vi "cursor window logic.vi"(4 "h. offset":dbl, 6 "CursIdx":i32, 7 "cursor window action":T1=enum."check", 8 "window":dbl=nan, 9 "center":dbl=nan, 10 "cursor bracket in":refnum<vi>, 11 "cursor bracket in":T2={"left"=2044.0881763527054, "right "=2126.7657992565055, "center"=2085.4269878046052, "window"=82.67762290380006, "cursors"=[], "relative"=0, "absolute"=0, "fixed vertical offset"=2421.6740576496672, "vertical offset"=2421.6740576496672, "skew"=2421.6740576496672, "default window frac"=2421.6740576496672, "kind"=enum."fancy", "skew.left"=2.0, "skew.right"=0.0, "Plot ref"=refnum, "wing order"=enum."back"}) -> (2 "reference out":refnum<vi>, 3 "cursor window out":T2={"left"=2044.0881763527054, "right "=2126.7657992565055, "center"=2085.4269878046052, "window"=82.67762290380006, "cursors"=[], "relative"=0, "absolute"=0, "fixed vertical offset"=2421.6740576496672, "vertical offset"=2421.6740576496672, "skew"=2421.6740576496672, "default window frac"=2421.6740576496672, "kind"=enum."fancy", "skew.left"=2.0, "skew.right"=0.0, "Plot ref"=refnum, "wing order"=enum."back"})   [LabVIEW 2014]
uses:
  cursor winow.ctl
  cursor window action.ctl
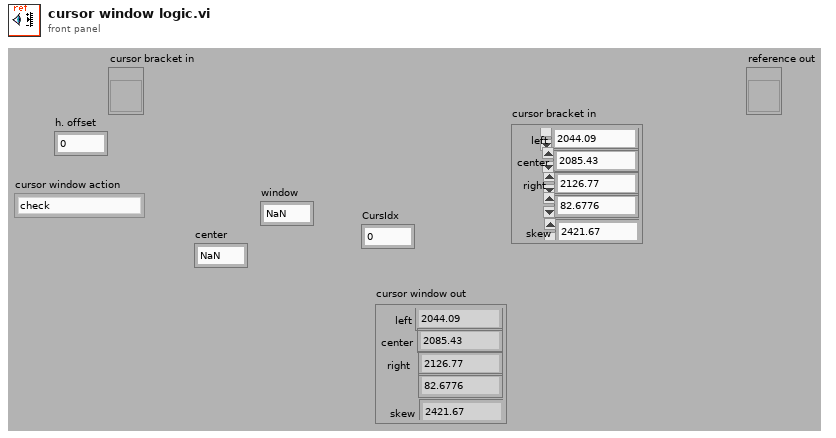
[diagram p1: front panel]
types:
  T1 = typedef "cursor window action.ctl" = enum16{"balance", "h. offset change", "cursor moves", "change center", "change window", "init", "check", "reset", "set y to middle", "idle", "-write all Y", "-write left.X", "-write center.X", "-write right.X", "-write all X", "-change center", "-change window", "-change skew", "-read cursor 2", "-read cursor 1", "-read cursor 0", "-read all cursors", "-reset", "-read plot scale", "-set y to middle", "-Q: center.Y is visible", "-Q: window is visible", "-parse center.Y", "-right left from center", "-left move", "-right move", "-set center.Y", "-empty", "-set cursors to default", "-check", "-write center.Y", "-copy cursor 1", "-copy cursor 0", "-copy cursor 2", "move right", "move left", "shrink", "broaden", "skew up", "skew down", "-write plot scale", "zoom X", "change cen&win", "zoom to all data"}
  T2 = typedef "cursor winow.ctl" = cluster{"left":dbl, "right ":dbl, "center":dbl, "window":dbl, "cursors":i32[], "relative":i32, "absolute":i32, "fixed vertical offset":dbl, "vertical offset":dbl, "skew":dbl, "default window frac":dbl, "kind":enum16{"symmetric", "skewed", "fancy"}, "skew.left":dbl, "skew.right":dbl, "Plot ref":refnum<vi>, "wing order":enum16{"forw", "back"}}
  T3 = cluster{"left":dbl, "right ":dbl, "center":dbl, "window":dbl, "cursors":i32[], "relative":i32, "absolute":i32, "fixed vertical offset":dbl, "vertical offset":dbl, "skew":dbl, "default window frac":dbl, "kind":enum16{"symmetric", "skewed", "fancy"}, "skew.left":dbl, "skew.right":dbl, "Plot ref":refnum<vi>, "wing order":enum16{"forw", "back"}}
  T4 = typedef "LVCursorListTypeDef.ctl" = cluster{"Name":string, "Color":u32, "Style":u8, "Point Style":u8, "Name Visible":bool, "Allow Drag":bool, "Cursor Mode":u32, "Plot":i32, "Index":i32, "Position":cluster{"X":dbl, "Y":dbl}, "X Scale":u32, "Y Scale":u32, "Watch Plots":i32[], "Watch All Plots":bool, "Plot Area":i32, "Label Offset":cluster{"X":dbl, "Y":dbl}}[]
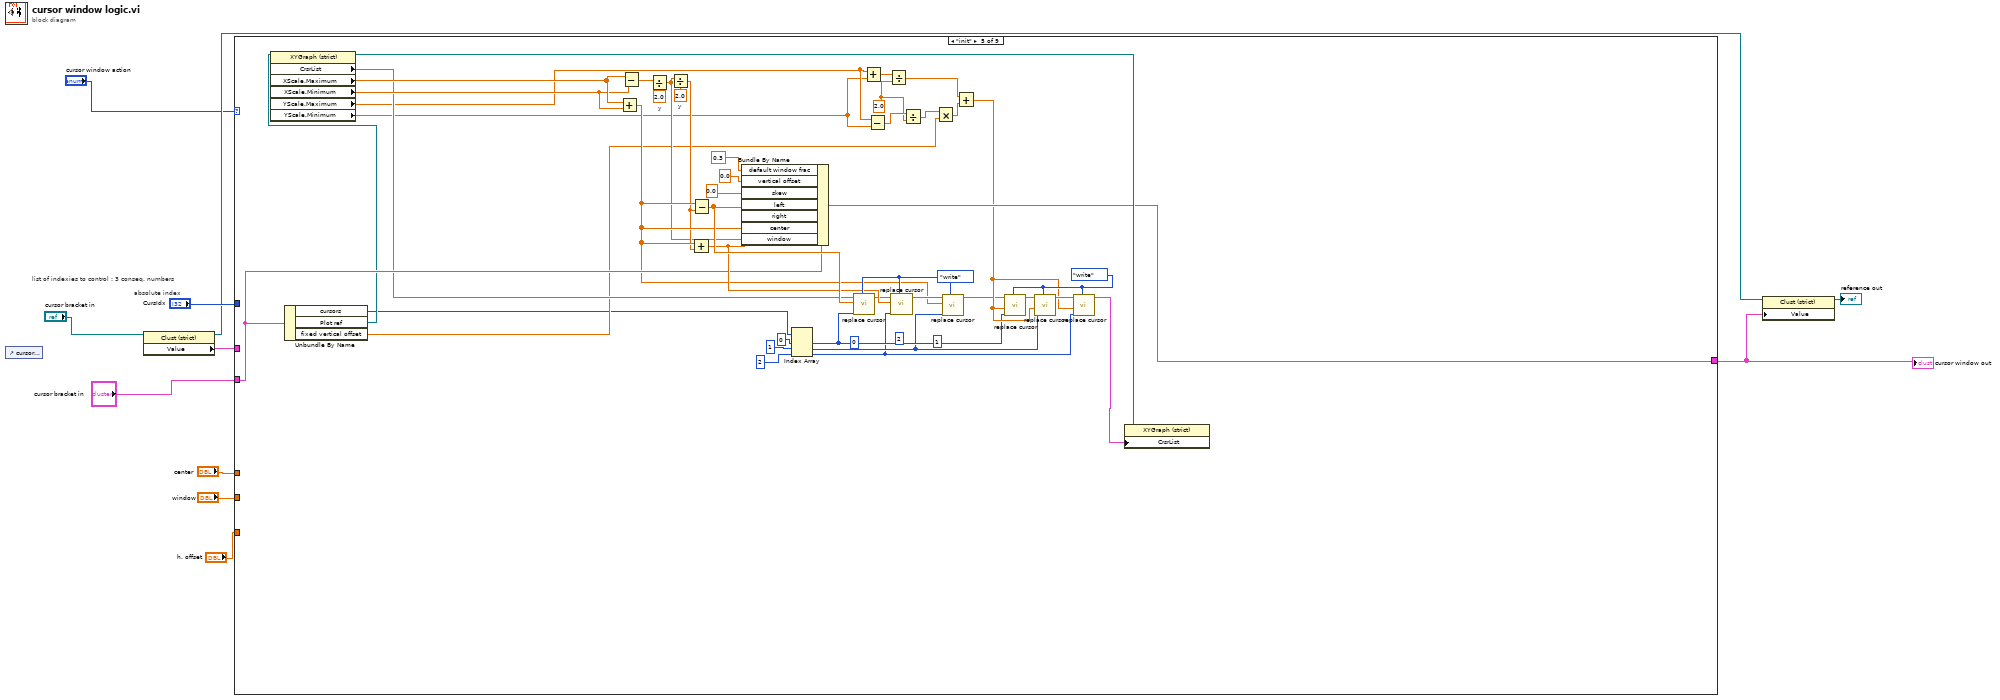
[diagram p0: block diagram]
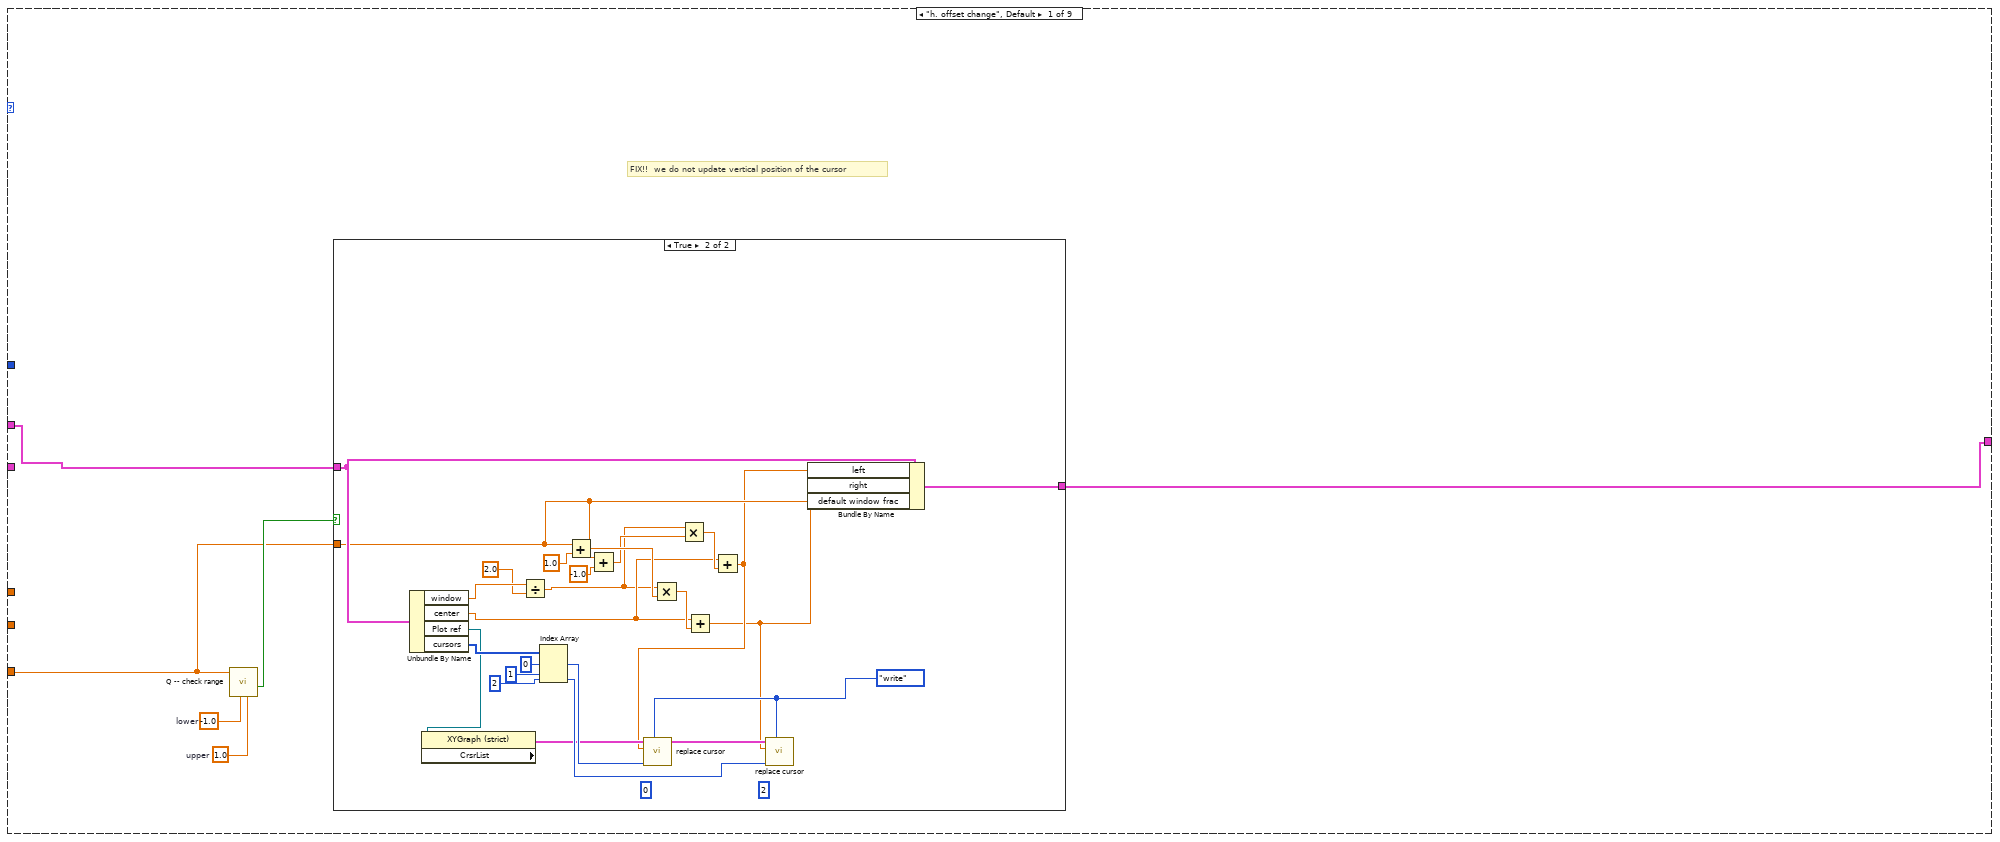
[diagram p2: hidden frame]
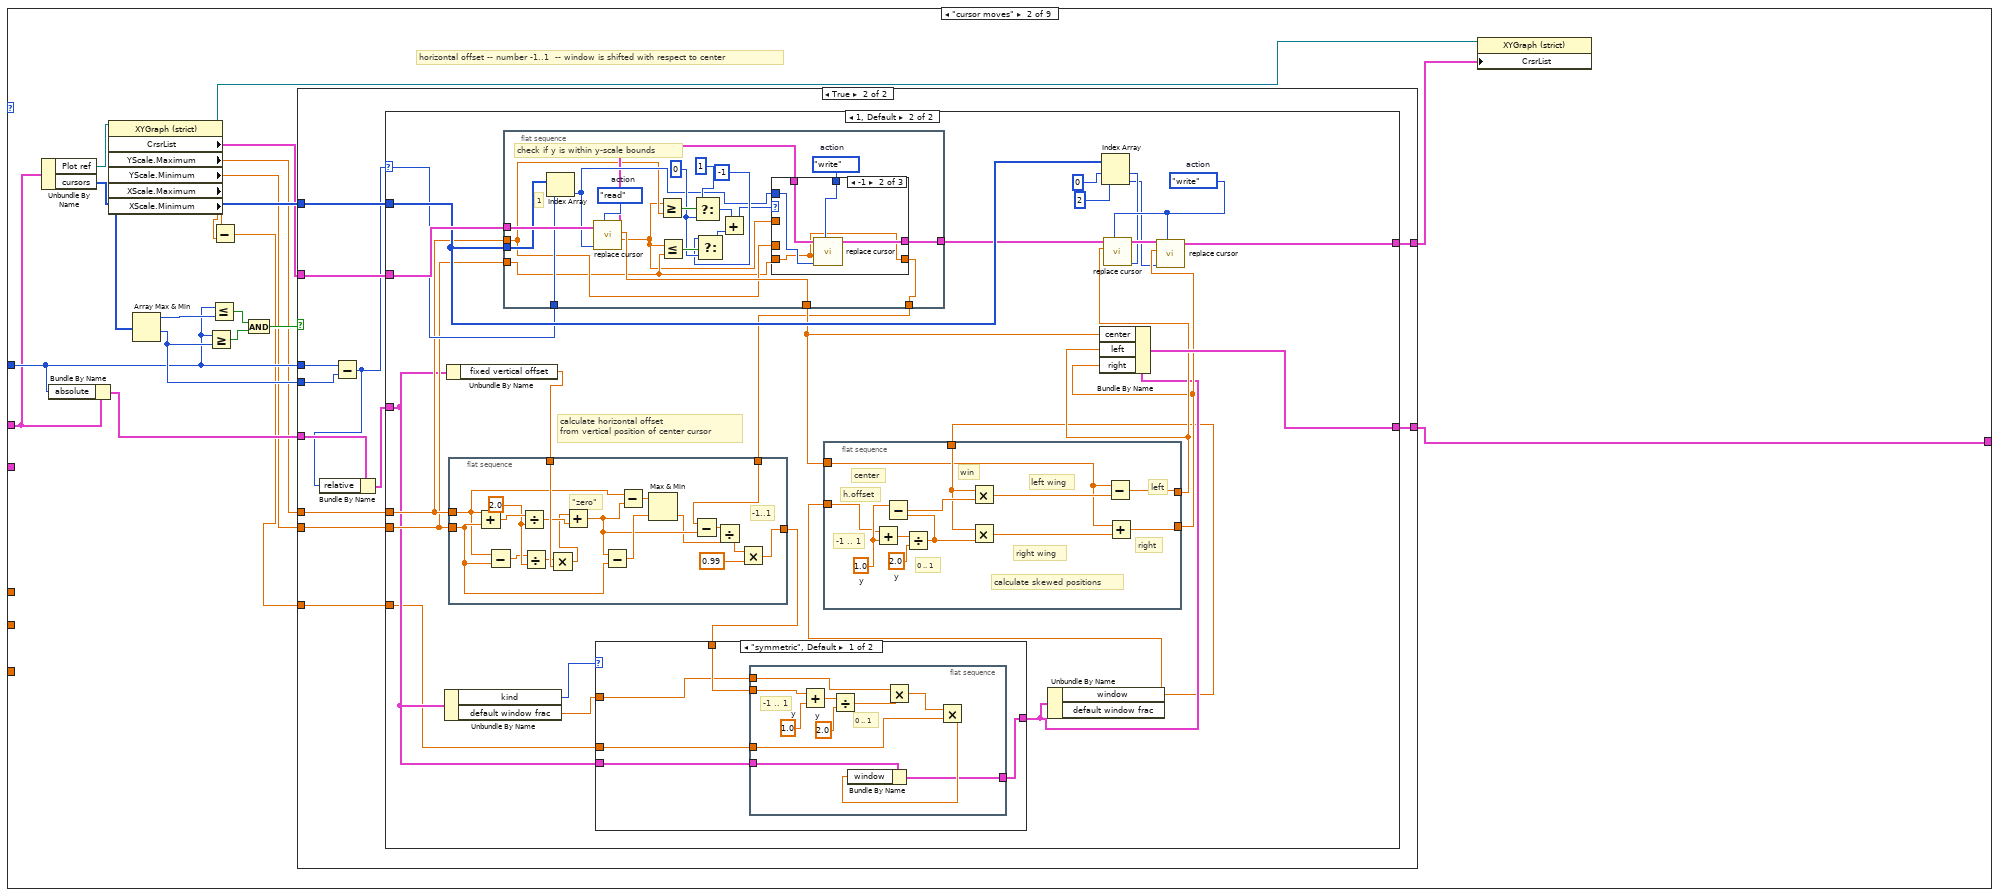
[diagram p4: hidden frame]
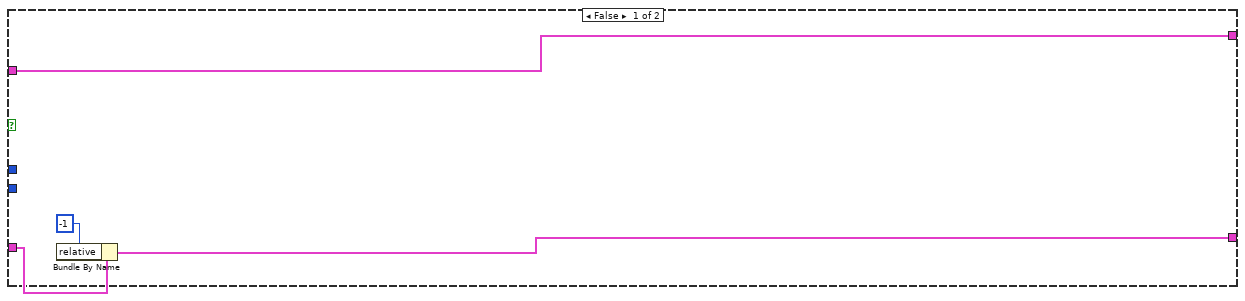
[diagram p5: hidden frame]
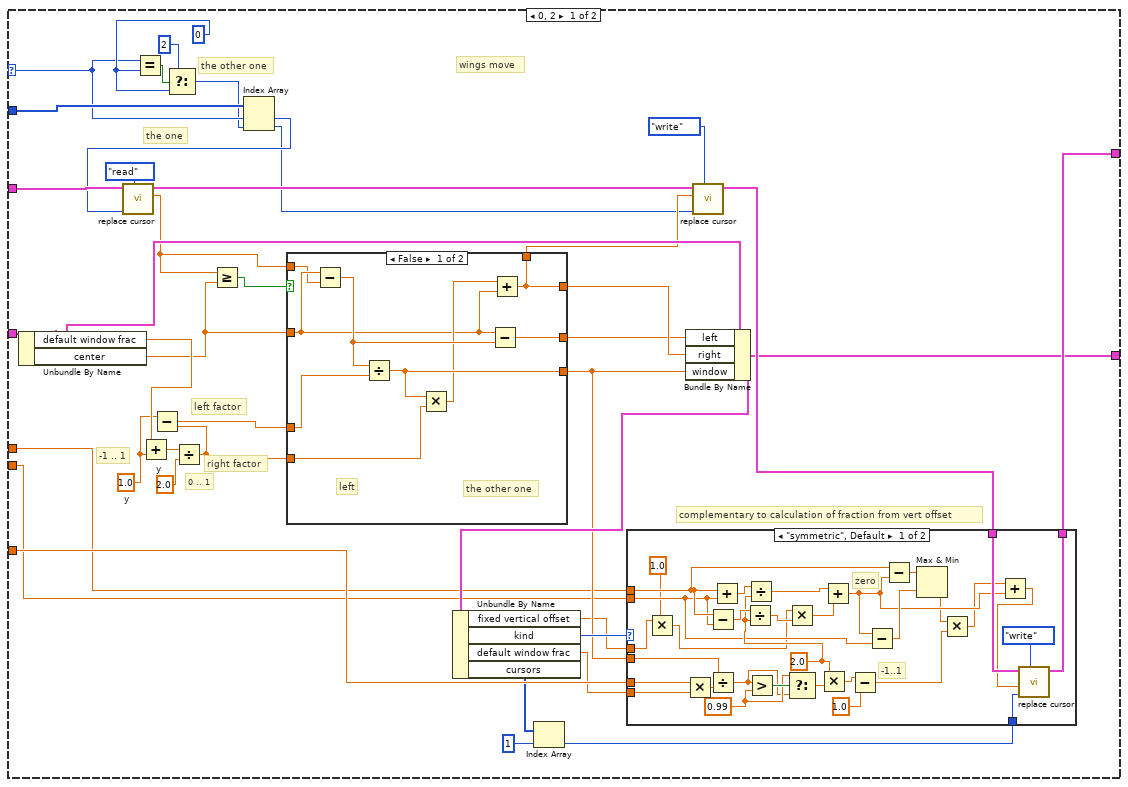
[diagram p6: hidden frame]
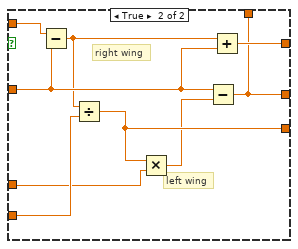
[diagram p8: hidden frame]
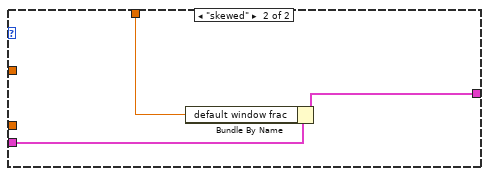
[diagram p9: hidden frame]
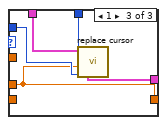
[diagram p11: hidden frame]
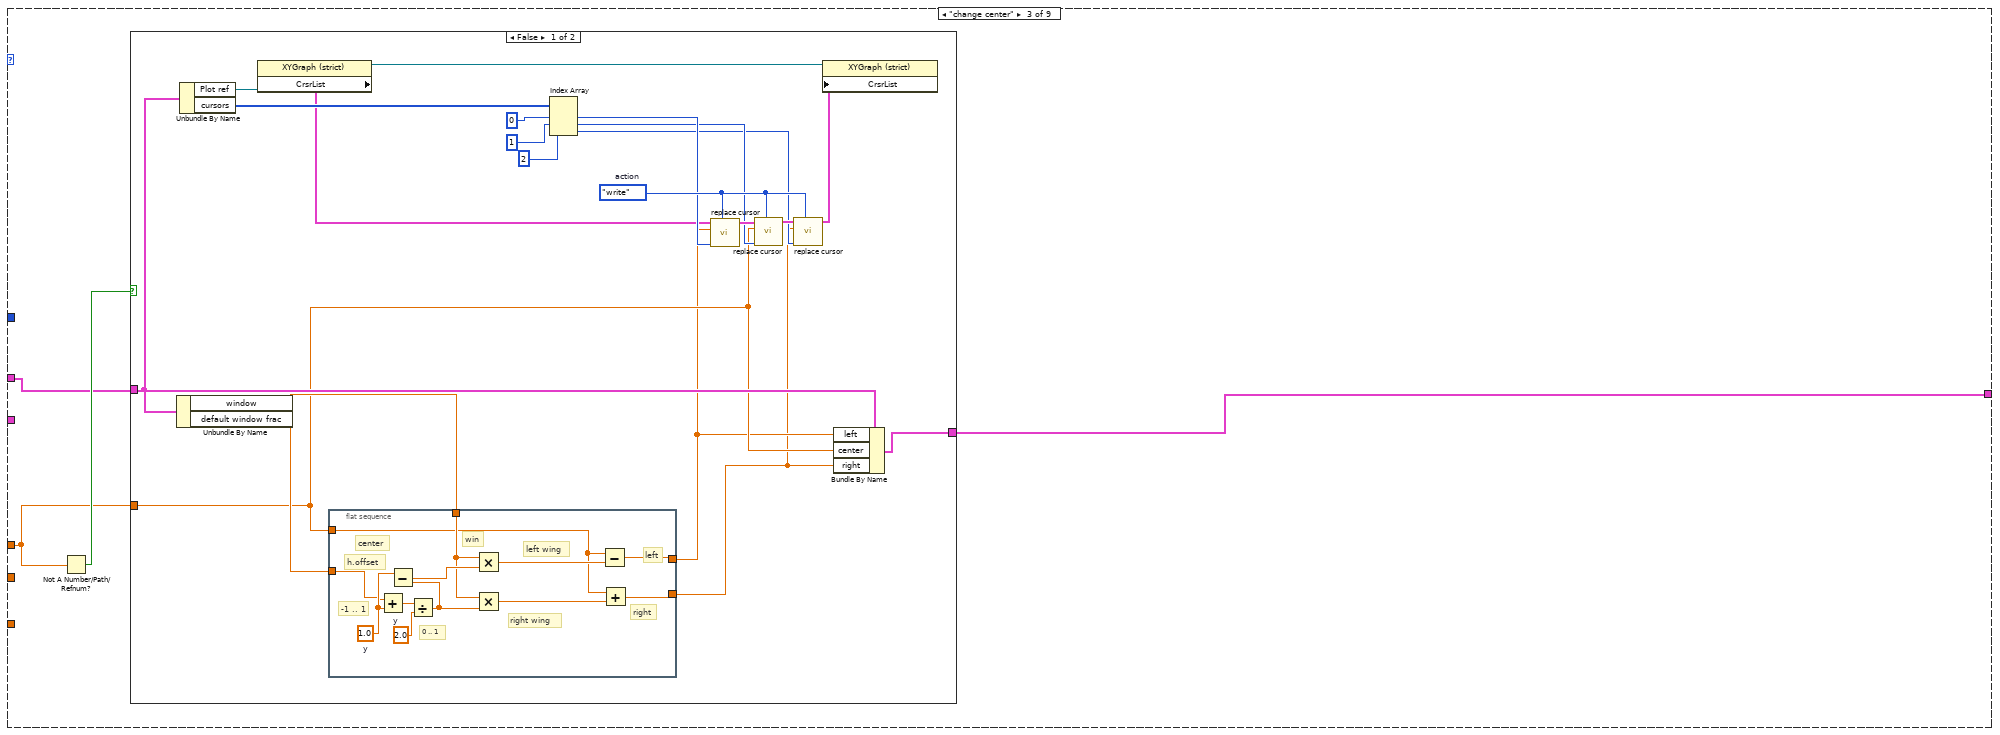
[diagram p12: hidden frame]
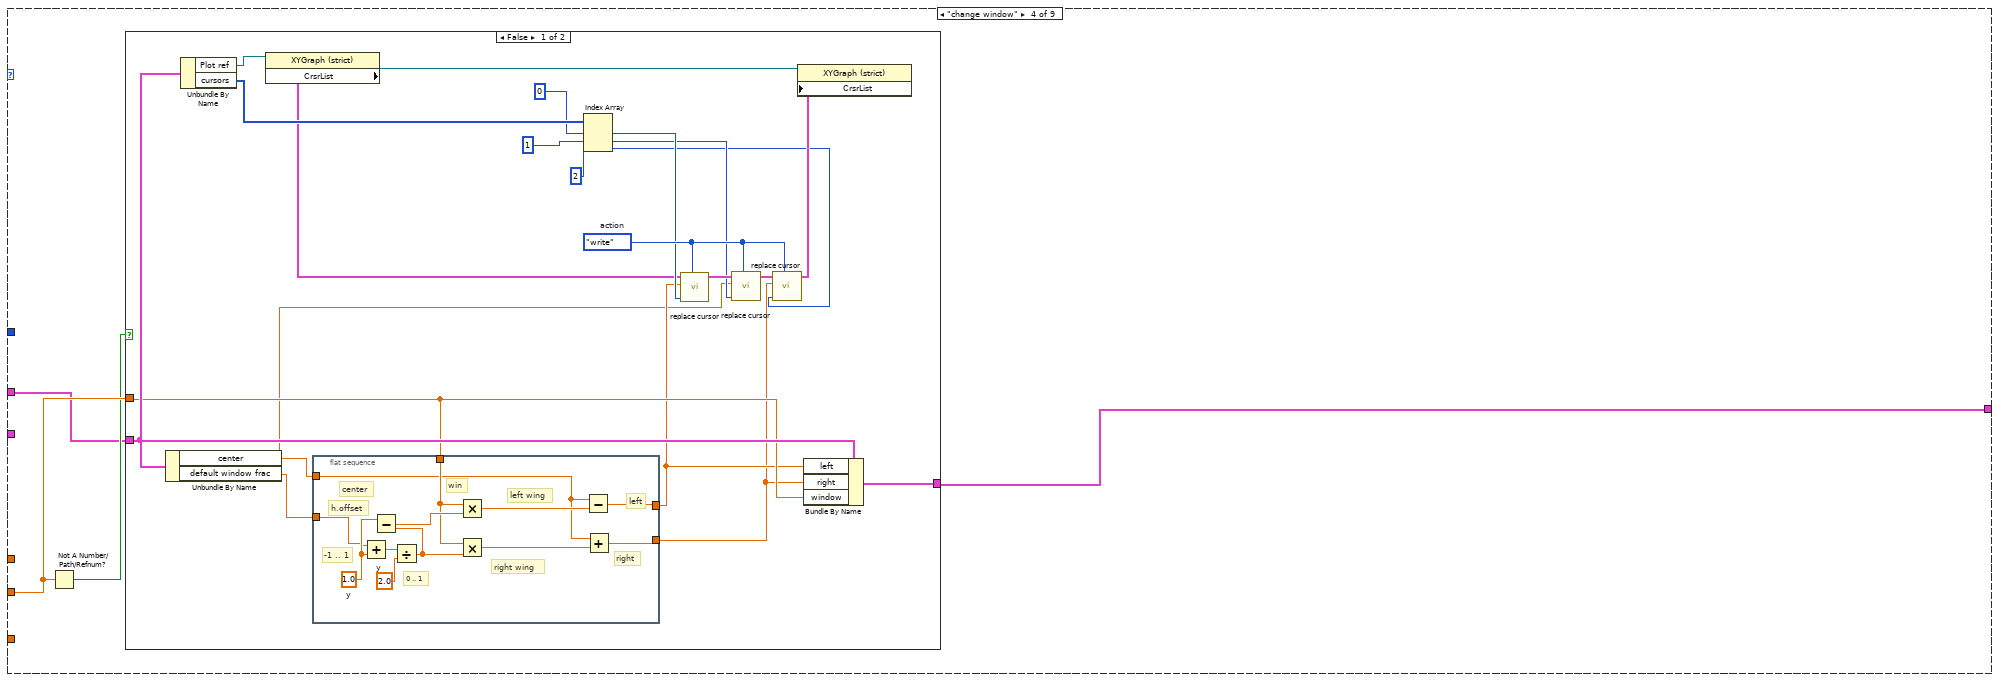
[diagram p14: hidden frame]
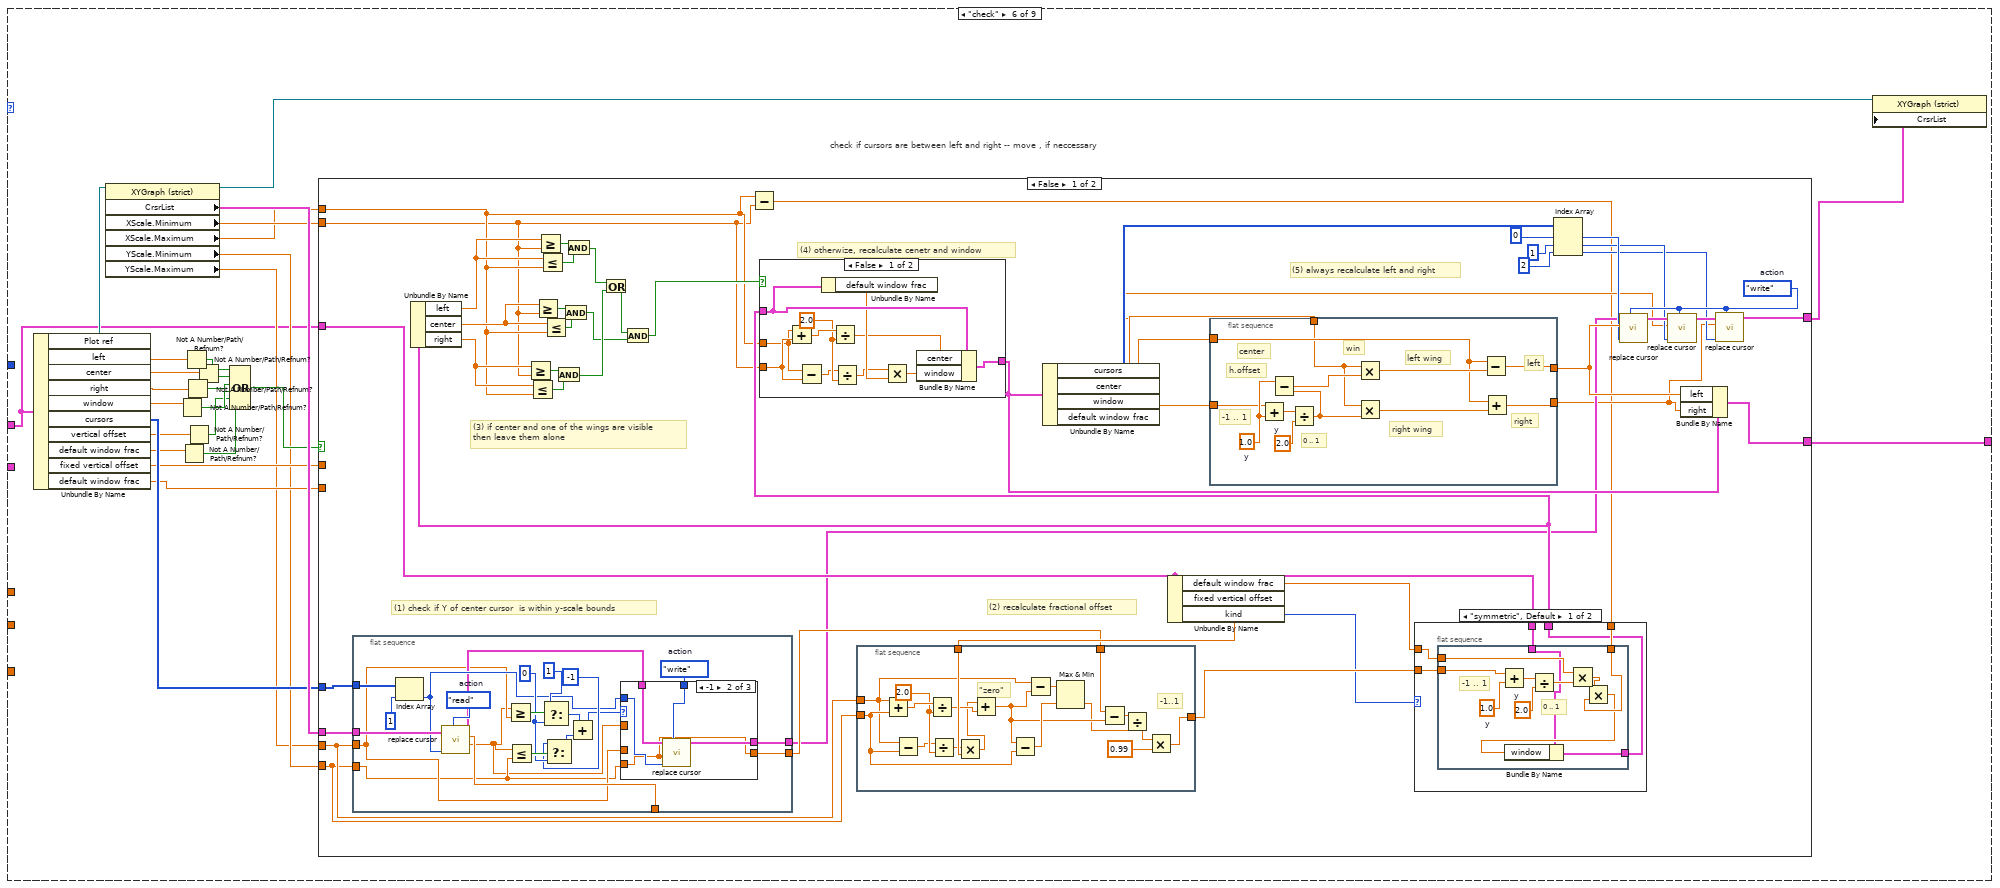
[diagram p16: hidden frame]
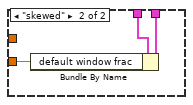
[diagram p17: hidden frame]
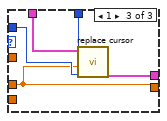
[diagram p19: hidden frame]
diagram:
  # "list of indexies to control : 3 conseq. numbers"
  # "absolute index"
  n1 = control-ref of="cursor bracket in"() -> ()  [unwired: 1 out]
  n2 = property class="Clust (strict)"(reference="cursor bracket in") -> (reference out=w6:refnum<vi>, "Value"=w7:T3)  [unwired: 1 in, 1 out]
  n3 = case shown="\"init\"" "cursor window action" {
    tunnel: "cursor bracket in" -> [_ _ _ _ w385 _ _ _ _]
    tunnel: [w12 w50 w280 w318 w386 w419 w605 w636 w661] -> w5
    tunnel: "CursIdx" -> [_ w56 _ _ _ _ _ _ _]
    tunnel: "center" -> [_ _ w278 _ _ _ _ _ _]
    tunnel: "window" -> [_ _ _ w317 _ _ _ _ _]
    tunnel: w7 -> [w17 w44 w277 w315 _ w396 w603 w636 w661]
    tunnel: "h. offset" -> [w13 _ _ _ _ _ _ _ _]
    frame "h. offset change", Default {
      w15 = 1.0  # upper
      w16 = -1.0  # lower
      # "FIX!!  we do not update vertical position of the cursor"
      n4 = call "Q -- check range.vi"("upper"=w15, "lower"=w16, "number"=w13) -> ("in range?"=w14:bool)  [unwired: 4 in, 4 out]
      n5 = case shown="True" w14 {
        tunnel: w17 -> [w18 w43]
        tunnel: w13 -> [_ w37]
        tunnel: [w18 w19] -> w12
        frame False {
        }
        frame True {
          w25 = enum16{"", "read", "write"}."write" ("Enum")
          (unwired) 2 ("cursor index")
          (unwired) 0 ("cursor index")
          n6 = Unbundle By Name(w43) -> ("window"=w42:dbl, "center"=w34:dbl, "Plot ref"=w23:refnum<vi>, "cursors"=w24:i32[])
          n7 = property class="XYGraph (strict)"(reference=w23) -> ("CrsrList"=w22:T4)  [unwired: 1 in, 2 out]
          n8 = Divide(x=w42, y=2.0) -> (x/y=w32:dbl)
          n9 = Index Array(array=w24, index #1=0 ("index"), index #2=1 ("index"), index #3=2 ("index")) -> (element #1=w28:i32, element #3=w27:i32)  [unwired: 1 out]
          n10 = Add(x=w37, y=1.0) -> (x+y=w36:dbl)
          n11 = Add(x=w37, y=-1.0) -> (x+y=w33:dbl)
          n12 = Multiply(x=w32, y=w36) -> (x*y=w40:dbl)
          n13 = Multiply(x=w32, y=w33) -> (x*y=w35:dbl)
          n14 = Add(x=w34, y=w40) -> (x+y=w20:dbl)
          n15 = Add(x=w34, y=w35) -> (x+y=w21:dbl)
          n16 = call "replace cursor.vi"("action"=w25, "cursor index"=w28, "new X"=w21, "Cursor List in"=w22) -> ("Cursor List Out"=w26:T4)  [unwired: 5 in, 2 out]
          n17 = call "replace cursor.vi"("action"=w25, "cursor index"=w27, "new X"=w20, "Cursor List in"=w26) -> ()  [unwired: 5 in, 3 out]
          n18 = Bundle By Name(cluster=w43, "left"=w21, "right"=w20, "default window frac"=w37) -> (w19:T3)
        }
      }
    }
    frame "cursor moves" {
      # "horizontal offset -- number -1..1  -- window is shifted with respect to center"
      n19 = Unbundle By Name(w44) -> ("Plot ref"=w54:refnum<vi>, "cursors"=w55:i32[])
      n20 = Bundle By Name(cluster=w44, "absolute"=w56) -> (w57:T3)
      n21 = property on="Property Node" class="XYGraph (strict)"(reference=w54) -> (reference out=w51:refnum<vi>, "CrsrList"=w53:T4, "YScale.Maximum"=w49:dbl, "YScale.Minimum"=w48:dbl, "XScale.Maximum"=w47:dbl, "XScale.Minimum"=w46:dbl)  [unwired: 1 in, 1 out]
      n22 = Array Max & Min(array=w55) -> (max value=w62:i32, min value=w58:i32)  [unwired: 2 out]
      n23 = Greater Or Equal?(x=w56, y=w58) -> (x >= y?=w61:bool)
      n24 = Less Or Equal?(x=w56, y=w62) -> (x <= y?=w60:bool)
      n25 = Subtract(x=w47, y=w46) -> (x-y=w45:dbl)
      n26 = And(x=w60, y=w61) -> (x .and. y?=w59:bool)
      n27 = case shown="True" w59 {
        tunnel: w57 -> [w65 w72]
        tunnel: [w63 w78] -> w50
        tunnel: w53 -> [w66 w77]
        tunnel: [w66 w76] -> w52
        tunnel: w55 -> [_ w75]
        tunnel: w56 -> [_ w74]
        tunnel: w58 -> [_ w73]
        tunnel: w49 -> [_ w69]
        tunnel: w48 -> [_ w68]
        tunnel: w45 -> [_ w67]
        frame False {
          n28 = Bundle By Name(cluster=w65, "relative"=-1) -> (w63:T3)
        }
        frame True {
          n29 = Subtract(x=w74, y=w73) -> (x-y=w70:i32)
          n30 = Bundle By Name(cluster=w72, "relative"=w70) -> (w71:T3)
          n31 = case shown="1, Default" w70 {
            selector: w70 -> [w97 w186]
            tunnel: w77 -> [w116 w194]
            tunnel: w71 -> [w114 w174]
            tunnel: [w88 w193] -> w78
            tunnel: [w91 w190] -> w76
            tunnel: w75 -> [w110 w187]
            tunnel: w69 -> [w84 w179]
            tunnel: w68 -> [w83 w177]
            tunnel: w67 -> [w89 w168]
            frame 0, 2 {
              w99 = 0 ("y")
              w106 = 1.0  # y
              w109 = 2.0  # y
              # "complementary to calculation of fraction from vert offset"
              # "wings move"
              # "the one"
              # "the other one"
              # "left factor"
              # "right factor"
              # "0 .. 1"
              # "-1 .. 1"
              n32 = Unbundle By Name(w114) -> ("default window frac"=w107:dbl, "center"=w95:dbl)
              n33 = Equal?(x=w97, y=w99) -> (x = y?=w98:bool)
              n34 = Add(x=w107, y=w106) -> (x+y=w108:dbl)
              n35 = Select(t=2, s=w98, f=w99) -> (s? t:f=w94:i32)
              n36 = Divide(x=w108, y=w109) -> (x/y=w104:dbl)
              n37 = Subtract(x=w106, y=w104) -> (x-y=w102:dbl)
              n38 = Index Array(array=w110, index #1=w97, index #2=w94) -> (element #1=w111:i32, element #2=w93:i32)
              n39 = call "replace cursor.vi"("action"=enum16{"", "read", "write"}."read", "cursor index"=w111, "Cursor List in"=w116) -> ("read X"=w92:dbl, "Cursor List Out"=w113:T4)  [unwired: 6 in, 1 out]
              n40 = Greater Or Equal?(x=w92, y=w95) -> (x >= y?=w105:bool)
              n41 = case shown="False" w105 {
                tunnel: w92 -> [w150 w167]
                tunnel: w104 -> [w156 w166]
                tunnel: [w157 w165] -> w85
                tunnel: [w152 w160] -> w103
                tunnel: w102 -> [w158 w164]
                tunnel: [w154 w159] -> w101
                tunnel: [w152 w159] -> w96
                tunnel: w95 -> [w151 w163]
                frame False {
                  # "left"
                  # "the other one"
                  n42 = Subtract(x=w151, y=w150) -> (x-y=w155:dbl)
                  n43 = Divide(x=w155, y=w158) -> (x/y=w157:dbl)
                  n44 = Multiply(x=w157, y=w156) -> (x*y=w153:dbl)
                  n45 = Subtract(x=w151, y=w155) -> (x-y=w154:dbl)
                  n46 = Add(x=w153, y=w151) -> (x+y=w152:dbl)
                }
                frame True {
                  # "right wing"
                  # "left wing"
                  n47 = Subtract(x=w167, y=w163) -> (x-y=w162:dbl)
                  n48 = Divide(x=w162, y=w166) -> (x/y=w165:dbl)
                  n49 = Multiply(x=w165, y=w164) -> (x*y=w161:dbl)
                  n50 = Subtract(x=w163, y=w161) -> (x-y=w159:dbl)
                  n51 = Add(x=w162, y=w163) -> (x+y=w160:dbl)
                }
              }
              n52 = Bundle By Name(cluster=w114, "left"=w101, "right"=w103, "window"=w85) -> (w88:T3)
              n53 = Unbundle By Name(w88) -> ("fixed vertical offset"=w82:dbl, "kind"=w87:enum16{"symmetric", "skewed", "fancy"}, "default window frac"=w86:dbl, "cursors"=w81:i32[])
              n54 = Index Array(array=w81, index=1) -> (element=w79:i32)
              n55 = call "replace cursor.vi"("action"=enum16{"", "read", "write"}."write", "cursor index"=w93, "new X"=w96, "Cursor List in"=w113) -> ("Cursor List Out"=w90:T4)  [unwired: 5 in, 2 out]
              n56 = case shown="\"symmetric\", Default" w87 {
                tunnel: [w133 w149] -> w91
                tunnel: w90 -> [w134 w149]
                tunnel: w89 -> [w148 _]
                tunnel: w86 -> [w119 _]
                tunnel: w85 -> [w131 _]
                tunnel: w84 -> [w127 _]
                tunnel: w83 -> [w126 _]
                tunnel: w82 -> [w118 _]
                tunnel: w79 -> [w132 _]
                frame "symmetric", Default {
                  w139 = 2.0 ("x")
                  w146 = 0.99 ("y")
                  # "zero"
                  # "-1..1"
                  n57 = Multiply(x=w118, y=1.0) -> (x*y=w117:dbl)
                  n58 = Multiply(x=w148, y=w119) -> (x*y=w130:dbl)
                  n59 = Subtract(x=w127, y=w126) -> (x-y=w140:dbl)
                  n60 = Divide(x=w131, y=w130) -> (x/y=w145:dbl)
                  n61 = Add(x=w127, y=w126) -> (x+y=w141:dbl)
                  n62 = Divide(x=w140, y=w139) -> (x/y=w136:dbl)
                  n63 = Divide(x=w141, y=w139) -> (x/y=w138:dbl)
                  n64 = Greater?(x=w145, y=w146) -> (0:w147:bool)
                  n65 = Multiply(x=w117, y=w136) -> (x*y=w137:dbl)
                  n66 = Select(t=w146, s=w147, f=w145) -> (s? t:f=w144:dbl)
                  n67 = Multiply(x=w139, y=w144) -> (x*y=w143:dbl)
                  n68 = Add(x=w138, y=w137) -> (x+y=w125:dbl)
                  n69 = Subtract(x=w143, y=1.0) -> (x-y=w123:dbl)
                  n70 = Subtract(x=w125, y=w126) -> (x-y=w128:dbl)
                  n71 = Subtract(x=w127, y=w125) -> (x-y=w129:dbl)
                  n72 = Max & Min(x=w129, y=w128) -> (min(x,y)=w124:dbl)  [unwired: 1 out]
                  n73 = Multiply(x=w124, y=w123) -> (x*y=w122:dbl)
                  n74 = Add(x=w122, y=w125) -> (x+y=w121:dbl)
                  n75 = call "replace cursor.vi"("action"=enum16{"", "read", "write"}."write", "cursor index"=w132, "new  Y"=w121, "Cursor List in"=w134) -> ("Cursor List Out"=w133:T4)  [unwired: 5 in, 2 out]
                }
                frame "skewed" {
                }
              }
            }
            frame 1, Default {
              w191 = enum16{"", "read", "write"}."write"  # action
              # "calculate horizontal offset\nfrom vertical position of center cursor"
              n76 = Unbundle By Name(w174) -> ("kind"=w175:enum16{"symmetric", "skewed", "fancy"}, "default window frac"=w169:dbl)
              n77 = Unbundle By Name(w174) -> ("fixed vertical offset"=w185:dbl)
              n78 = flat-sequence {
                tunnel: w179 -> [w263]
                tunnel: w185 -> [w273]
                tunnel: w177 -> [w269]
                tunnel: [w261] -> w173
                tunnel: w176 -> [w259]
                frame #0 {
                  w275 = 2.0 ("y")
                  # "-1..1"
                  # "\"zero\""
                  n79 = Add(x=w263, y=w269) -> (x+y=w276:dbl)
                  n80 = Subtract(x=w263, y=w269) -> (x-y=w274:dbl)
                  n81 = Divide(x=w276, y=w275) -> (x/y=w271:dbl)
                  n82 = Divide(x=w274, y=w275) -> (x/y=w272:dbl)
                  n83 = Multiply(x=w272, y=w273) -> (x*y=w270:dbl)
                  n84 = Add(x=w270, y=w271) -> (x+y=w266:dbl)
                  n85 = Subtract(x=w266, y=w269) -> (x-y=w267:dbl)
                  n86 = Subtract(x=w263, y=w266) -> (x-y=w268:dbl)
                  n87 = Max & Min(x=w268, y=w267) -> (min(x,y)=w264:dbl)  [unwired: 1 out]
                  n88 = Subtract(x=w259, y=w266) -> (x-y=w265:dbl)
                  n89 = Divide(x=w265, y=w264) -> (x/y=w262:dbl)
                  n90 = Multiply(x=w262, y=0.99) -> (x*y=w261:dbl)
                }
              }
              n91 = flat-sequence {
                tunnel: w194 -> [w234]
                tunnel: w187 -> [w232]
                tunnel: w186 -> [w231]
                tunnel: [w230] -> w184
                tunnel: w179 -> [w219]
                tunnel: [w218] -> w178
                tunnel: w177 -> [w217]
                tunnel: [w215] -> w176
                frame #0 {
                  w216 = enum16{"", "read", "write"}."write"  # action
                  w227 = 0
                  w233 = enum16{"", "read", "write"}."read"  # action
                  # "check if y is within y-scale bounds"
                  # "1"
                  n92 = Index Array(array=w232, index=w231) -> (element=w221:i32)
                  n93 = call "replace cursor.vi"("action"=w233, "cursor index"=w221, "Cursor List in"=w234) -> ("read Y"=w214:dbl, "read X"=w230:dbl, "Cursor List Out"=w220:T4)  [unwired: 6 in]
                  n94 = Greater Or Equal?(x=w214, y=w219) -> (x >= y?=w229:bool)
                  n95 = Less Or Equal?(x=w214, y=w217) -> (x <= y?=w228:bool)
                  n96 = Select(t=1 ("index"), s=w229, f=w227) -> (s? t:f=w223:i32)
                  n97 = Select(t=-1 ("index"), s=w228, f=w227) -> (s? t:f=w224:i32)
                  n98 = Add(x=w223, y=w224) -> (x+y=w222:i32)
                  n99 = case shown="-1" w222 {
                    tunnel: w221 -> [_ w241 w246]
                    tunnel: w220 -> [w236 w240 w245]
                    tunnel: w219 -> [_ _ w242]
                    tunnel: [w236 w239 w244] -> w218
                    tunnel: w217 -> [_ w237 _]
                    tunnel: w216 -> [_ w238 w243]
                    tunnel: [w235 w237 w242] -> w215
                    tunnel: w214 -> [w235 _ _]
                    frame 0, Default {
                    }
                    frame -1 {
                      n100 = call "replace cursor.vi"("action"=w238, "cursor index"=w241, "new  Y"=w237, "Cursor List in"=w240) -> ("Cursor List Out"=w239:T4)  [unwired: 5 in, 2 out]
                    }
                    frame 1 {
                      n101 = call "replace cursor.vi"("action"=w243, "cursor index"=w246, "new  Y"=w242, "Cursor List in"=w245) -> ("Cursor List Out"=w244:T4)  [unwired: 5 in, 2 out]
                    }
                  }
                }
              }
              n102 = case shown="\"symmetric\", Default" w175 {
                tunnel: w174 -> [w197 w213]
                tunnel: [w196 w212] -> w171
                tunnel: w173 -> [w199 w211]
                tunnel: w169 -> [w198 _]
                tunnel: w168 -> [w195 _]
                frame "symmetric", Default {
                  n103 = flat-sequence {
                    tunnel: w199 -> [w207]
                    tunnel: w198 -> [w205]
                    tunnel: w195 -> [w203]
                    tunnel: w197 -> [w201]
                    tunnel: [w200] -> w196
                    frame #0 {
                      w208 = 1.0  # y
                      w210 = 2.0  # y
                      # "0 .. 1"
                      # "-1 .. 1"
                      n104 = Add(x=w207, y=w208) -> (x+y=w209:dbl)
                      n105 = Divide(x=w209, y=w210) -> (x/y=w206:dbl)
                      n106 = Multiply(x=w205, y=w206) -> (x*y=w204:dbl)
                      n107 = Multiply(x=w204, y=w203) -> (x*y=w202:dbl)
                      n108 = Bundle By Name(cluster=w201, "window"=w202) -> (w200:T3)
                    }
                  }
                }
                frame "skewed" {
                  n109 = Bundle By Name(cluster=w213, "default window frac"=w211) -> (w212:T3)
                }
              }
              n110 = flat-sequence {
                tunnel: w172 -> [w251]
                tunnel: w170 -> [w250]
                tunnel: w184 -> [w249]
                tunnel: [w248] -> w183
                tunnel: [w247] -> w182
                frame #0 {
                  w256 = 1.0  # y
                  w258 = 2.0  # y
                  # "calculate skewed positions"
                  # "right"
                  # "left"
                  # "win"
                  # "h.offset"
                  # "center"
                  # "left wing"
                  # "right wing"
                  # "0 .. 1"
                  # "-1 .. 1"
                  n111 = Add(x=w251, y=w256) -> (x+y=w257:dbl)
                  n112 = Divide(x=w257, y=w258) -> (x/y=w253:dbl)
                  n113 = Subtract(x=w256, y=w253) -> (x-y=w252:dbl)
                  n114 = Multiply(x=w250, y=w252) -> (x*y=w255:dbl)
                  n115 = Multiply(x=w250, y=w253) -> (x*y=w254:dbl)
                  n116 = Subtract(x=w249, y=w255) -> (x-y=w248:dbl)
                  n117 = Add(x=w249, y=w254) -> (x+y=w247:dbl)
                }
              }
              n118 = Unbundle By Name(w171) -> ("window"=w170:dbl, "default window frac"=w172:dbl)
              n119 = Bundle By Name(cluster=w171, "center"=w184, "left"=w183, "right"=w182) -> (w193:T3)
              n120 = Index Array(array=w187, index #1=0 ("cursor index"), index #2=2 ("index")) -> (element #1=w188:i32, element #2=w181:i32)
              n121 = call "replace cursor.vi"("action"=w191, "cursor index"=w188, "new X"=w183, "Cursor List in"=w178) -> ("Cursor List Out"=w192:T4)  [unwired: 5 in, 2 out]
              n122 = call "replace cursor.vi"("action"=w191, "cursor index"=w181, "new X"=w182, "Cursor List in"=w192) -> ("Cursor List Out"=w190:T4)  [unwired: 5 in, 2 out]
            }
          }
        }
      }
      n123 = property on="Property Node" class="XYGraph (strict)"(reference=w51, "CrsrList"=w52) -> ()  [unwired: 1 in, 2 out]
    }
    frame "change center" {
      n124 = Not A Number/Path/Refnum?(number/path/refnum=w278) -> (NaN/Path/Refnum?=w279:bool)
      n125 = case shown="False" w279 {
        tunnel: w277 -> [w297 w314]
        tunnel: [w291 w314] -> w280
        tunnel: w278 -> [w283 _]
        frame False {
          w299 = enum16{"", "read", "write"}."write"  # action
          n126 = Unbundle By Name(w297) -> ("window"=w289:dbl, "default window frac"=w290:dbl)
          n127 = Unbundle By Name(w297) -> ("Plot ref"=w295:refnum<vi>, "cursors"=w296:i32[])
          n128 = property on="Property Node" class="XYGraph (strict)"(reference=w295) -> (reference out=w292:refnum<vi>, "CrsrList"=w294:T4)  [unwired: 1 in, 1 out]
          n129 = flat-sequence {
            tunnel: w290 -> [w306]
            tunnel: w289 -> [w305]
            tunnel: w283 -> [w304]
            tunnel: [w303] -> w282
            tunnel: [w302] -> w281
            frame #0 {
              w311 = 1.0  # y
              w313 = 2.0  # y
              # "right"
              # "left"
              # "win"
              # "h.offset"
              # "center"
              # "left wing"
              # "right wing"
              # "0 .. 1"
              # "-1 .. 1"
              n130 = Add(x=w306, y=w311) -> (x+y=w312:dbl)
              n131 = Divide(x=w312, y=w313) -> (x/y=w308:dbl)
              n132 = Subtract(x=w311, y=w308) -> (x-y=w307:dbl)
              n133 = Multiply(x=w305, y=w307) -> (x*y=w310:dbl)
              n134 = Multiply(x=w305, y=w308) -> (x*y=w309:dbl)
              n135 = Subtract(x=w304, y=w310) -> (x-y=w303:dbl)
              n136 = Add(x=w304, y=w309) -> (x+y=w302:dbl)
            }
          }
          n137 = Index Array(array=w296, index #1=0 ("cursor index"), index #2=1 ("cursor index"), index #3=2 ("cursor index")) -> (element #1=w298:i32, element #2=w286:i32, element #3=w284:i32)
          n138 = call "replace cursor.vi"("action"=w299, "cursor index"=w298, "new X"=w282, "Cursor List in"=w294) -> ("Cursor List Out"=w301:T4)  [unwired: 5 in, 2 out]
          n139 = call "replace cursor.vi"("action"=w299, "cursor index"=w286, "new X"=w283, "Cursor List in"=w301) -> ("Cursor List Out"=w300:T4)  [unwired: 5 in, 2 out]
          n140 = call "replace cursor.vi"("action"=w299, "cursor index"=w284, "new X"=w281, "Cursor List in"=w300) -> ("Cursor List Out"=w293:T4)  [unwired: 5 in, 2 out]
          n141 = property on="Property Node" class="XYGraph (strict)"(reference=w292, "CrsrList"=w293) -> ()  [unwired: 1 in, 2 out]
          n142 = Bundle By Name(cluster=w297, "left"=w282, "center"=w283, "right"=w281) -> (w291:T3)
        }
        frame True {
        }
      }
    }
    frame "change window" {
      n143 = Not A Number/Path/Refnum?(number/path/refnum=w317) -> (NaN/Path/Refnum?=w316:bool)
      n144 = case shown="False" w316 {
        tunnel: w317 -> [w322 _]
        tunnel: w315 -> [w335 w352]
        tunnel: [w329 w352] -> w318
        frame False {
          w337 = enum16{"", "read", "write"}."write"  # action
          n145 = Unbundle By Name(w335) -> ("center"=w319:dbl, "default window frac"=w323:dbl)
          n146 = Unbundle By Name(w335) -> ("Plot ref"=w333:refnum<vi>, "cursors"=w334:i32[])
          n147 = property on="Property Node" class="XYGraph (strict)"(reference=w333) -> (reference out=w330:refnum<vi>, "CrsrList"=w332:T4)  [unwired: 1 in, 1 out]
          n148 = flat-sequence {
            tunnel: w323 -> [w344]
            tunnel: w322 -> [w343]
            tunnel: w319 -> [w342]
            tunnel: [w341] -> w321
            tunnel: [w340] -> w320
            frame #0 {
              w349 = 1.0  # y
              w351 = 2.0  # y
              # "right"
              # "left"
              # "win"
              # "h.offset"
              # "center"
              # "left wing"
              # "right wing"
              # "0 .. 1"
              # "-1 .. 1"
              n149 = Add(x=w344, y=w349) -> (x+y=w350:dbl)
              n150 = Divide(x=w350, y=w351) -> (x/y=w346:dbl)
              n151 = Subtract(x=w349, y=w346) -> (x-y=w345:dbl)
              n152 = Multiply(x=w343, y=w345) -> (x*y=w348:dbl)
              n153 = Multiply(x=w343, y=w346) -> (x*y=w347:dbl)
              n154 = Subtract(x=w342, y=w348) -> (x-y=w341:dbl)
              n155 = Add(x=w342, y=w347) -> (x+y=w340:dbl)
            }
          }
          n156 = Index Array(array=w334, index #1=0 ("index"), index #2=1 ("index"), index #3=2 ("index")) -> (element #1=w336:i32, element #2=w325:i32, element #3=w324:i32)
          n157 = call "replace cursor.vi"("action"=w337, "cursor index"=w336, "new X"=w321, "Cursor List in"=w332) -> ("Cursor List Out"=w339:T4)  [unwired: 5 in, 2 out]
          n158 = call "replace cursor.vi"("action"=w337, "cursor index"=w325, "new X"=w319, "Cursor List in"=w339) -> ("Cursor List Out"=w338:T4)  [unwired: 5 in, 2 out]
          n159 = call "replace cursor.vi"("action"=w337, "cursor index"=w324, "new X"=w320, "Cursor List in"=w338) -> ("Cursor List Out"=w331:T4)  [unwired: 5 in, 2 out]
          n160 = property on="Property Node" class="XYGraph (strict)"(reference=w330, "CrsrList"=w331) -> ()  [unwired: 1 in, 2 out]
          n161 = Bundle By Name(cluster=w335, "left"=w321, "right"=w320, "window"=w322) -> (w329:T3)
        }
        frame True {
        }
      }
    }
    frame "init" {
      w369 = enum16{"", "read", "write"}."write" ("Enum")
      w372 = 2.0 ("y")
      w378 = 2.0  # y
      w381 = 2.0  # y
      (unwired) 1 ("cursor index")
      w395 = enum16{"", "read", "write"}."write" ("Enum")
      (unwired) 2 ("cursor index")
      (unwired) 0 ("cursor index")
      n162 = Unbundle By Name(w385) -> ("cursors"=w361:i32[], "Plot ref"=w384:refnum<vi>, "fixed vertical offset"=w362:dbl)
      n163 = property on="Property Node" class="XYGraph (strict)"(reference=w384) -> (reference out=w387:refnum<vi>, "CrsrList"=w375:T4, "XScale.Maximum"=w383:dbl, "XScale.Minimum"=w382:dbl, "YScale.Maximum"=w364:dbl, "YScale.Minimum"=w363:dbl)  [unwired: 1 in, 1 out]
      n164 = Add(x=w383, y=w382) -> (x+y=w379:dbl)
      n165 = Subtract(x=w383, y=w382) -> (x-y=w380:dbl)
      n166 = Divide(x=w380, y=w381) -> (x/y=w376:dbl)
      n167 = Divide(x=w376, y=w378) -> (x/y=w377:dbl)
      n168 = Add(x=w379, y=w377) -> (x+y=w392:dbl)
      n169 = Subtract(x=w379, y=w377) -> (x-y=w393:dbl)
      n170 = Bundle By Name(cluster=w385, "default window frac"=0.3, "vertical offset"=0.0, "skew"=0.0, "left"=w393, "right"=w392, "center"=w379, "window"=w376) -> (w386:T2)
      n171 = Index Array(array=w361, index #1=0 ("index"), index #2=1 ("index"), index #3=2 ("index")) -> (element #1=w359:i32, element #2=w358:i32, element #3=w357:i32)
      n172 = call "replace cursor.vi"("action"=w395, "cursor index"=w359, "new X"=w393, "Cursor List in"=w375) -> ("Cursor List Out"=w388:T4)  [unwired: 5 in, 2 out]
      n173 = Add(x=w364, y=w363) -> (x+y=w374:dbl)
      n174 = Subtract(x=w364, y=w363) -> (x-y=w373:dbl)
      n175 = Divide(x=w374, y=w372) -> (x/y=w366:dbl)
      n176 = call "replace cursor.vi"("action"=w395, "cursor index"=w357, "new X"=w392, "Cursor List in"=w388) -> ("Cursor List Out"=w394:T4)  [unwired: 5 in, 2 out]
      n177 = Divide(x=w373, y=w372) -> (x/y=w368:dbl)
      n178 = Multiply(x=w368, y=w362) -> (x*y=w367:dbl)
      n179 = call "replace cursor.vi"("action"=w395, "cursor index"=w358, "new X"=w379, "Cursor List in"=w394) -> ("Cursor List Out"=w356:T4)  [unwired: 5 in, 2 out]
      n180 = Add(x=w366, y=w367) -> (x+y=w365:dbl)
      n181 = call "replace cursor.vi"("action"=w369, "cursor index"=w359, "new  Y"=w365, "Cursor List in"=w356) -> ("Cursor List Out"=w370:T4)  [unwired: 5 in, 2 out]
      n182 = call "replace cursor.vi"("action"=w369, "cursor index"=w358, "new  Y"=w365, "Cursor List in"=w370) -> ("Cursor List Out"=w371:T4)  [unwired: 5 in, 2 out]
      n183 = call "replace cursor.vi"("action"=w369, "cursor index"=w357, "new  Y"=w365, "Cursor List in"=w371) -> ("Cursor List Out"=w355:T4)  [unwired: 5 in, 2 out]
      n184 = property on="Property Node" class="XYGraph (strict)"(reference=w387, "CrsrList"=w355) -> ()  [unwired: 1 in, 2 out]
    }
    frame "check" {
      # "check if cursors are between left and right -- move , if neccessary"
      n185 = Unbundle By Name(w396) -> ("Plot ref"=w416:refnum<vi>, "left"=w413:dbl, "center"=w412:dbl, "right"=w414:dbl, "window"=w415:dbl, "cursors"=w406:i32[], "vertical offset"=w405:dbl, "default window frac"=w404:dbl, "fixed vertical offset"=w400:dbl, "default window frac"=w401:dbl)
      n186 = property on="Property Node" class="XYGraph (strict)"(reference=w416) -> (reference out=w420:refnum<vi>, "CrsrList"=w421:T4, "XScale.Minimum"=w418:dbl, "XScale.Maximum"=w417:dbl, "YScale.Minimum"=w399:dbl, "YScale.Maximum"=w398:dbl)  [unwired: 1 in, 1 out]
      n187 = Not A Number/Path/Refnum?(number/path/refnum=w415) -> (NaN/Path/Refnum?=w408:bool)
      n188 = Not A Number/Path/Refnum?(number/path/refnum=w404) -> (NaN/Path/Refnum?=w403:bool)
      n189 = Not A Number/Path/Refnum?(number/path/refnum=w413) -> (NaN/Path/Refnum?=w411:bool)
      n190 = Not A Number/Path/Refnum?(number/path/refnum=w414) -> (NaN/Path/Refnum?=w409:bool)
      n191 = Not A Number/Path/Refnum?(number/path/refnum=w405) -> (NaN/Path/Refnum?=w402:bool)
      n192 = Not A Number/Path/Refnum?(number/path/refnum=w412) -> (NaN/Path/Refnum?=w410:bool)
      n193 = Compound Arithmetic op=OR(w411, w410, w409, w408, w402, w403) -> (w407:bool)
      n194 = case shown="False" w407 {
        tunnel: w401 -> [_ w583]
        tunnel: w396 -> [w452 w589]
        tunnel: w421 -> [w459 w596]
        tunnel: [w437 w568] -> w397
        tunnel: [w441 w588] -> w419
        tunnel: w418 -> [w423 w591]
        tunnel: w417 -> [w424 w590]
        tunnel: w406 -> [w460 w597]
        tunnel: w400 -> [_ w572]
        tunnel: w399 -> [w456 w571]
        tunnel: w398 -> [w457 w570]
        frame False {
          w436 = enum16{"", "read", "write"}."write"  # action
          # "(3) if center and one of the wings are visible \nthen leave them alone"
          # "(4) otherwize, recalculate cenetr and window"
          # "(5) always recalculate left and right"
          # "(2) recalculate fractional offset"
          # "(1) check if Y of center cursor  is within y-scale bounds"
          n195 = flat-sequence {
            tunnel: w459 -> [w538]
            tunnel: w460 -> [w536]
            tunnel: [w535] -> _
            tunnel: w457 -> [w524]
            tunnel: [w523] -> w443
            tunnel: w456 -> [w522]
            tunnel: [w520] -> w454
            frame #0 {
              w521 = enum16{"", "read", "write"}."write"  # action
              w532 = 0
              w537 = enum16{"", "read", "write"}."read"  # action
              n196 = Index Array(array=w536, index=1) -> (element=w526:i32)
              n197 = call "replace cursor.vi"("action"=w537, "cursor index"=w526, "Cursor List in"=w538) -> ("read Y"=w519:dbl, "read X"=w535:dbl, "Cursor List Out"=w525:T4)  [unwired: 6 in]
              n198 = Greater Or Equal?(x=w519, y=w524) -> (x >= y?=w534:bool)
              n199 = Less Or Equal?(x=w519, y=w522) -> (x <= y?=w533:bool)
              n200 = Select(t=1 ("index"), s=w534, f=w532) -> (s? t:f=w528:i32)
              n201 = Select(t=-1 ("index"), s=w533, f=w532) -> (s? t:f=w529:i32)
              n202 = Add(x=w528, y=w529) -> (x+y=w527:i32)
              n203 = case shown="-1" w527 {
                tunnel: w526 -> [_ w545 w550]
                tunnel: w525 -> [w540 w544 w549]
                tunnel: w524 -> [_ _ w546]
                tunnel: [w540 w543 w548] -> w523
                tunnel: w522 -> [_ w541 _]
                tunnel: w521 -> [_ w542 w547]
                tunnel: [w539 w541 w546] -> w520
                tunnel: w519 -> [w539 _ _]
                frame 0, Default {
                }
                frame -1 {
                  n204 = call "replace cursor.vi"("action"=w542, "cursor index"=w545, "new  Y"=w541, "Cursor List in"=w544) -> ("Cursor List Out"=w543:T4)  [unwired: 5 in, 2 out]
                }
                frame 1 {
                  n205 = call "replace cursor.vi"("action"=w547, "cursor index"=w550, "new  Y"=w546, "Cursor List in"=w549) -> ("Cursor List Out"=w548:T4)  [unwired: 5 in, 2 out]
                }
              }
            }
          }
          n206 = Subtract(x=w424, y=w423) -> (x-y=w422:dbl)
          n207 = flat-sequence {
            tunnel: w457 -> [w504]
            tunnel: w455 -> [w514]
            tunnel: w456 -> [w510]
            tunnel: [w502] -> w453
            tunnel: w454 -> [w500]
            frame #0 {
              w516 = 2.0 ("y")
              # "-1..1"
              # "\"zero\""
              n208 = Add(x=w504, y=w510) -> (x+y=w517:dbl)
              n209 = Subtract(x=w504, y=w510) -> (x-y=w515:dbl)
              n210 = Divide(x=w517, y=w516) -> (x/y=w512:dbl)
              n211 = Divide(x=w515, y=w516) -> (x/y=w513:dbl)
              n212 = Multiply(x=w513, y=w514) -> (x*y=w511:dbl)
              n213 = Add(x=w511, y=w512) -> (x+y=w507:dbl)
              n214 = Subtract(x=w507, y=w510) -> (x-y=w508:dbl)
              n215 = Subtract(x=w504, y=w507) -> (x-y=w509:dbl)
              n216 = Max & Min(x=w509, y=w508) -> (min(x,y)=w505:dbl)  [unwired: 1 out]
              n217 = Subtract(x=w500, y=w507) -> (x-y=w506:dbl)
              n218 = Divide(x=w506, y=w505) -> (x/y=w503:dbl)
              n219 = Multiply(x=w503, y=0.99) -> (x*y=w502:dbl)
            }
          }
          n220 = Unbundle By Name(w452) -> ("default window frac"=w425:dbl, "fixed vertical offset"=w455:dbl, "kind"=w426:enum16{"symmetric", "skewed", "fancy"})
          n221 = flat-sequence {
            tunnel: w427 -> [w492]
            tunnel: [w491] -> w450
            tunnel: [w490] -> w433
            tunnel: w445 -> [w489]
            tunnel: w446 -> [w488]
            frame #0 {
              w497 = 1.0  # y
              w499 = 2.0  # y
              # "right"
              # "left"
              # "win"
              # "h.offset"
              # "center"
              # "left wing"
              # "right wing"
              # "0 .. 1"
              # "-1 .. 1"
              n222 = Add(x=w488, y=w497) -> (x+y=w498:dbl)
              n223 = Divide(x=w498, y=w499) -> (x/y=w494:dbl)
              n224 = Subtract(x=w497, y=w494) -> (x-y=w493:dbl)
              n225 = Multiply(x=w489, y=w493) -> (x*y=w496:dbl)
              n226 = Multiply(x=w489, y=w494) -> (x*y=w495:dbl)
              n227 = Subtract(x=w492, y=w496) -> (x-y=w491:dbl)
              n228 = Add(x=w492, y=w495) -> (x+y=w490:dbl)
            }
          }
          n229 = case shown="\"symmetric\", Default" w426 {
            tunnel: w453 -> [w473 w487]
            tunnel: w452 -> [w470 w486]
            tunnel: [w469 w485] -> w451
            tunnel: w425 -> [w472 _]
            tunnel: w422 -> [w471 _]
            frame "symmetric", Default {
              n230 = flat-sequence {
                tunnel: w473 -> [w481]
                tunnel: w472 -> [w479]
                tunnel: w471 -> [w477]
                tunnel: w470 -> [w475]
                tunnel: [w474] -> w469
                frame #0 {
                  w482 = 1.0  # y
                  w484 = 2.0  # y
                  # "0 .. 1"
                  # "-1 .. 1"
                  n231 = Add(x=w481, y=w482) -> (x+y=w483:dbl)
                  n232 = Divide(x=w483, y=w484) -> (x/y=w480:dbl)
                  n233 = Multiply(x=w479, y=w480) -> (x*y=w478:dbl)
                  n234 = Multiply(x=w478, y=w477) -> (x*y=w476:dbl)
                  n235 = Bundle By Name(cluster=w475, "window"=w476) -> (w474:T3)
                }
              }
            }
            frame "skewed" {
              n236 = Bundle By Name(cluster=w486, "default window frac"=w487) -> (w485:T3)
            }
          }
          n237 = Unbundle By Name(w451) -> ("left"=w466:dbl, "center"=w458:dbl, "right"=w461:dbl)
          n238 = Greater Or Equal?(x=w461, y=w423) -> (x >= y?=w463:bool)
          n239 = Less Or Equal?(x=w461, y=w424) -> (x <= y?=w462:bool)
          n240 = Greater Or Equal?(x=w458, y=w423) -> (x >= y?=w465:bool)
          n241 = Greater Or Equal?(x=w466, y=w423) -> (x >= y?=w468:bool)
          n242 = Less Or Equal?(x=w466, y=w424) -> (x <= y?=w467:bool)
          n243 = Less Or Equal?(x=w458, y=w424) -> (x <= y?=w464:bool)
          n244 = And(x=w463, y=w462) -> (x .and. y?=w431:bool)
          n245 = And(x=w465, y=w464) -> (x .and. y?=w429:bool)
          n246 = And(x=w468, y=w467) -> (x .and. y?=w432:bool)
          n247 = Or(x=w432, y=w431) -> (x .or. y?=w430:bool)
          n248 = And(x=w430, y=w429) -> (x .and. y?=w428:bool)
          n249 = case shown="False" w428 {
            tunnel: w423 -> [w556 _]
            tunnel: w424 -> [w555 _]
            tunnel: w451 -> [w560 w562]
            tunnel: [w561 w562] -> w444
            frame False {
              w558 = 2.0 ("y")
              n250 = Add(x=w555, y=w556) -> (x+y=w559:dbl)
              n251 = Subtract(x=w555, y=w556) -> (x-y=w557:dbl)
              n252 = Unbundle By Name(w560) -> ("default window frac"=w554:dbl)
              n253 = Divide(x=w559, y=w558) -> (x/y=w551:dbl)
              n254 = Divide(x=w557, y=w558) -> (x/y=w553:dbl)
              n255 = Multiply(x=w553, y=w554) -> (x*y=w552:dbl)
              n256 = Bundle By Name(cluster=w560, "center"=w551, "window"=w552) -> (w561:T3)
            }
            frame True {
            }
          }
          n257 = Unbundle By Name(w444) -> ("cursors"=w442:i32[], "center"=w427:dbl, "window"=w445:dbl, "default window frac"=w446:dbl)
          n258 = Index Array(array=w442, index #1=0, index #2=1, index #3=2) -> (element #1=w449:i32, element #2=w435:i32, element #3=w434:i32)
          n259 = call "replace cursor.vi"("action"=w436, "cursor index"=w449, "new X"=w450, "Cursor List in"=w443) -> ("Cursor List Out"=w447:T4)  [unwired: 5 in, 2 out]
          n260 = call "replace cursor.vi"("action"=w436, "cursor index"=w435, "new X"=w427, "Cursor List in"=w447) -> ("Cursor List Out"=w438:T4)  [unwired: 5 in, 2 out]
          n261 = Bundle By Name(cluster=w444, "left"=w450, "right"=w433) -> (w441:T3)
          n262 = call "replace cursor.vi"("action"=w436, "cursor index"=w434, "new X"=w433, "Cursor List in"=w438) -> ("Cursor List Out"=w437:T4)  [unwired: 5 in, 2 out]
        }
        frame True {
          w563 = 2.0 ("y")
          w593 = 2.0  # y
          (unwired) 1 ("cursor index")
          w567 = enum16{"", "read", "write"}."write" ("Enum")
          (unwired) 2 ("cursor index")
          (unwired) 0 ("cursor index")
          n263 = Add(x=w590, y=w591) -> (x+y=w592:dbl)
          n264 = Subtract(x=w590, y=w591) -> (x-y=w584:dbl)
          n265 = Index Array(array=w597, index #1=0 ("index"), index #2=1 ("index"), index #3=2 ("index")) -> (element #1=w566:i32, element #2=w564:i32, element #3=w565:i32)
          n266 = Divide(x=w592, y=w593) -> (x/y=w585:dbl)
          n267 = Multiply(x=w583, y=w584) -> (x*y=w582:dbl)
          n268 = Divide(x=w582, y=2.0) -> (x/y=w594:dbl)
          n269 = Subtract(x=w585, y=w594) -> (x-y=w587:dbl)
          n270 = call "replace cursor.vi"("action"=w567, "cursor index"=w566, "new X"=w587, "Cursor List in"=w596) -> ("Cursor List Out"=w598:T4)  [unwired: 5 in, 2 out]
          n271 = Add(x=w585, y=w594) -> (x+y=w586:dbl)
          n272 = call "replace cursor.vi"("action"=w567, "cursor index"=w565, "new X"=w586, "Cursor List in"=w598) -> ("Cursor List Out"=w602:T4)  [unwired: 5 in, 2 out]
          n273 = Bundle By Name(cluster=w589, "left"=w587, "right"=w586, "center"=w585, "window"=w582, "default window frac"=0.0 ("horizontal offset")) -> (w588:T3)
          n274 = call "replace cursor.vi"("action"=w567, "cursor index"=w564, "new X"=w585, "Cursor List in"=w602) -> ("Cursor List Out"=w569:T4)  [unwired: 5 in, 2 out]
          n275 = Subtract(x=w571, y=w570) -> (x-y=w575:dbl)
          n276 = Add(x=w570, y=w571) -> (x+y=w574:dbl)
          n277 = Divide(x=w574, y=w563) -> (x/y=w580:dbl)
          n278 = Divide(x=w575, y=w563) -> (x/y=w578:dbl)
          n279 = Multiply(x=w578, y=w572) -> (x*y=w579:dbl)
          n280 = Add(x=w580, y=w579) -> (x+y=w581:dbl)
          n281 = call "replace cursor.vi"("action"=w567, "cursor index"=w566, "new  Y"=w581, "Cursor List in"=w569) -> ("Cursor List Out"=w577:T4)  [unwired: 5 in, 2 out]
          n282 = call "replace cursor.vi"("action"=w567, "cursor index"=w564, "new  Y"=w581, "Cursor List in"=w577) -> ("Cursor List Out"=w576:T4)  [unwired: 5 in, 2 out]
          n283 = call "replace cursor.vi"("action"=w567, "cursor index"=w565, "new  Y"=w581, "Cursor List in"=w576) -> ("Cursor List Out"=w568:T4)  [unwired: 5 in, 2 out]
        }
      }
      n284 = property on="Property Node" class="XYGraph (strict)"(reference=w420, "CrsrList"=w397) -> ()  [unwired: 1 in, 2 out]
    }
    frame "reset" {
      w604 = 0.0
      (unwired) 1 ("cursor index")
      w625 = enum16{"", "read", "write"}."write" ("Enum")
      (unwired) 2 ("cursor index")
      (unwired) 0 ("cursor index")
      w628 = 2.0  # x
      w635 = enum16{"", "read", "write"}."read" ("Enum")
      # "THIS DOES NOT WORK \n\nFOR NOW"
      # "keep center the same \nmove braket cursors"
      n285 = Unbundle By Name(w603) -> ("Plot ref"=w607:refnum<vi>, "cursors"=w606:i32[])
      n286 = property on="Property Node" class="XYGraph (strict)"(reference=w607) -> (reference out=w609:refnum<vi>, "CrsrList"=w610:T4)  [unwired: 1 in, 1 out]
      n287 = Index Array(array=w606, index #1=0 ("index"), index #2=1 ("index"), index #3=2 ("index")) -> (element #1=w618:i32, element #2=w616:i32, element #3=w617:i32)
      n288 = call "replace cursor.vi"("action"=w635, "cursor index"=w618, "Cursor List in"=w610) -> ("read X"=w631:dbl, "Cursor List Out"=w613:T4)  [unwired: 6 in, 1 out]
      n289 = call "replace cursor.vi"("action"=w635, "cursor index"=w617, "Cursor List in"=w613) -> ("read X"=w634:dbl, "Cursor List Out"=w612:T4)  [unwired: 6 in, 1 out]
      n290 = call "replace cursor.vi"("action"=w635, "cursor index"=w616, "Cursor List in"=w612) -> ("read X"=w615:dbl, "Cursor List Out"=w611:T4)  [unwired: 6 in, 1 out]
      n291 = Subtract(x=w631, y=w615) -> (x-y=w632:dbl)
      n292 = Subtract(x=w634, y=w615) -> (x-y=w633:dbl)
      n293 = Absolute Value(x=w632) -> (abs(x)=w629:dbl)
      n294 = Absolute Value(x=w633) -> (abs(x)=w630:dbl)
      n295 = Max & Min(x=w630, y=w629) -> (min(x,y)=w626:dbl)  [unwired: 1 out]
      n296 = Multiply(x=w628, y=w626) -> (x*y=w627:dbl)
      n297 = Add(x=w615, y=w626) -> (x+y=w622:dbl)
      n298 = Subtract(x=w615, y=w626) -> (x-y=w623:dbl)
      n299 = call "replace cursor.vi"("action"=w625, "cursor index"=w618, "new X"=w623, "Cursor List in"=w611) -> ("Cursor List Out"=w614:T4)  [unwired: 5 in, 2 out]
      n300 = call "replace cursor.vi"("action"=w625, "cursor index"=w617, "new X"=w622, "Cursor List in"=w614) -> ("Cursor List Out"=w624:T4)  [unwired: 5 in, 2 out]
      n301 = call "replace cursor.vi"("action"=w625, "cursor index"=w616, "new X"=w615, "Cursor List in"=w624) -> ("Cursor List Out"=w608:T4)  [unwired: 5 in, 2 out]
      n302 = property on="Property Node" class="XYGraph (strict)"(reference=w609, "CrsrList"=w608) -> ()  [unwired: 1 in, 2 out]
      n303 = Bundle By Name(cluster=w603, "left"=w623, "right"=w622, "center"=w615, "window"=w627, "vertical offset"=w604, "default window frac"=w604) -> (w605:T3)
    }
    frame "set y to middle" {
      w644 = 2.0 ("y")
      (unwired) 1 ("cursor index")
      w647 = enum16{"", "read", "write"}."write" ("Enum")
      (unwired) 2 ("cursor index")
      (unwired) 0 ("cursor index")
      # "THIS DOES NOT WORK \n\nFOR NOW"
      n304 = Unbundle By Name(w636) -> ("fixed vertical offset"=w638:dbl, "Plot ref"=w651:refnum<vi>, "cursors"=w650:i32[])
      n305 = property on="Property Node" class="XYGraph (strict)"(reference=w651) -> (reference out=w652:refnum<vi>, "CrsrList"=w648:T4, "YScale.Maximum"=w639:dbl, "YScale.Minimum"=w640:dbl)  [unwired: 1 in, 1 out]
      n306 = Index Array(array=w650, index #1=0 ("index"), index #2=1 ("index"), index #3=2 ("index")) -> (element #1=w656:i32, element #2=w654:i32, element #3=w655:i32)
      n307 = Add(x=w639, y=w640) -> (x+y=w646:dbl)
      n308 = Subtract(x=w639, y=w640) -> (x-y=w645:dbl)
      n309 = Divide(x=w646, y=w644) -> (x/y=w641:dbl)
      n310 = Divide(x=w645, y=w644) -> (x/y=w643:dbl)
      n311 = Multiply(x=w643, y=w638) -> (x*y=w642:dbl)
      n312 = Add(x=w641, y=w642) -> (x+y=w637:dbl)
      n313 = call "replace cursor.vi"("action"=w647, "cursor index"=w656, "new  Y"=w637, "Cursor List in"=w648) -> ("Cursor List Out"=w653:T4)  [unwired: 5 in, 2 out]
      n314 = call "replace cursor.vi"("action"=w647, "cursor index"=w655, "new  Y"=w637, "Cursor List in"=w653) -> ("Cursor List Out"=w660:T4)  [unwired: 5 in, 2 out]
      n315 = call "replace cursor.vi"("action"=w647, "cursor index"=w654, "new  Y"=w637, "Cursor List in"=w660) -> ("Cursor List Out"=w649:T4)  [unwired: 5 in, 2 out]
      n316 = property on="Property Node" class="XYGraph (strict)"(reference=w652, "CrsrList"=w649) -> ()  [unwired: 1 in, 2 out]
    }
    frame "balance" {
    }
  }
  "cursor window out" <- w5
  n317 = property class="Clust (strict)"(reference=w6, "Value"=w5) -> (reference out=→"reference out":refnum<vi>)  [unwired: 1 in, 1 out]
